vi "ConvertWriteDataToReg.vi"(0 "SharedData Write":T1) -> (4 "registers to write":u16[](array[numeric]))   [LabVIEW 2019, in "ModbusSp.lvclass"]
uses:
  ModbusSp.lvclass
  WriteData.ctl
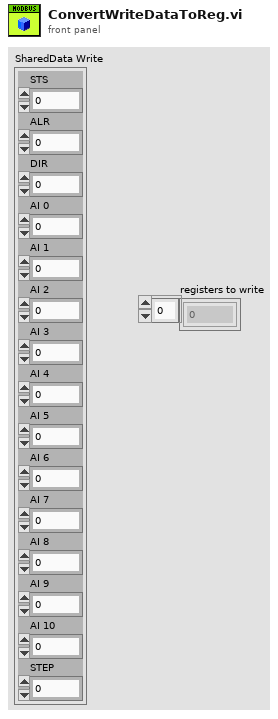
[diagram p1: front panel]
types:
  T1 = typedef "ModbusSp.lvclass/WriteData.ctl" = cluster{"STS":u16, "ALR":u16, "DIR":u16, "AI 0":sgl, "AI 1":sgl, "AI 2":sgl, "AI 3":sgl, "AI 4":sgl, "AI 5":sgl, "AI 6":sgl, "AI 7":sgl, "AI 8":sgl, "AI 9":sgl, "AI 10":sgl, "STEP":u16}
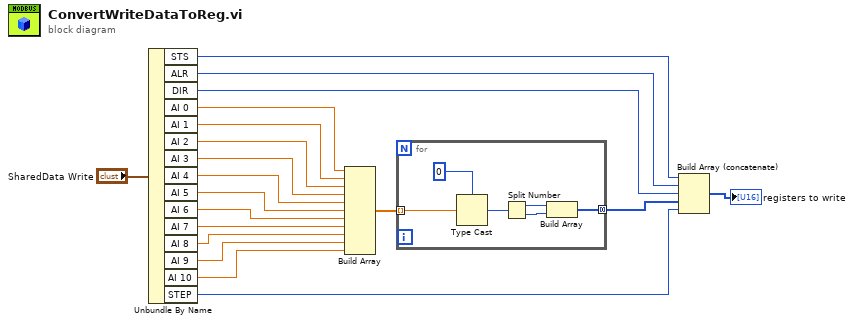
[diagram p0: block diagram]
diagram:
  n1 = Unbundle By Name("SharedData Write") -> ("STS"=w2:u16, "ALR"=w3:u16, "DIR"=w4:u16, "AI 0"=w17:sgl, "AI 1"=w16:sgl, "AI 2"=w15:sgl, "AI 3"=w14:sgl, "AI 4"=w13:sgl, "AI 5"=w12:sgl, "AI 6"=w11:sgl, "AI 7"=w10:sgl, "AI 8"=w9:sgl, "AI 9"=w8:sgl, "AI 10"=w7:sgl, "STEP"=w1:u16)
  n2 = Build Array(w17, w16, w15, w14, w13, w12, w11, w10, w9, w8, w7) -> (w6:sgl[])
  n3 = for {
    tunnel: w6 -> [w23] mode=indexing
    tunnel: [w20] -> w5 mode=concatenating
    n4 = Type Cast(type=u32 0, x=w23) -> (*(type *) &x=w25:u32)
    n5 = Split Number(x=w25) -> (hi(x)=w22:u16, lo(x)=w21:u16)
    n6 = Build Array(w22, w21) -> (w20:u16[])
  }
  n7 = Build Array (concatenate)(w2, w3, w4, w5, w1) -> (→"registers to write":u16[])
